vi "Event_LoadOrCreateRefs.vi"(8 "Error In":errorcluster) -> (0 "Error Out":errorcluster, 3 "HSE-Event":T1)   [LabVIEW 2014, in "hse-misc.lvlib"]
doc: "Returns the refnum of the HSE-Event\n\n\n\n____\nHAMPEL SOFTWARE ENGINEERING v0.7.0 (2018-07-16 18:12)"
uses:
  hse-misc.lvlib
  Event_GenericReference.ctl
  Event_GenericDatatype.ctl
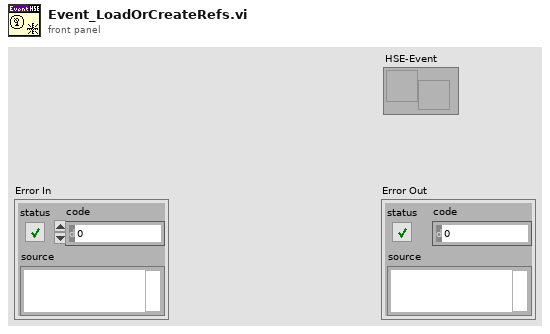
[diagram p1: front panel]
types:
  T1 = typedef "hse-misc.lvlib/Event_GenericReference.ctl" = refnum<user-event>
  T2 = typedef "hse-misc.lvlib/Event_GenericDatatype.ctl" = cluster{"name":string, "parameters":string, "data":variant}
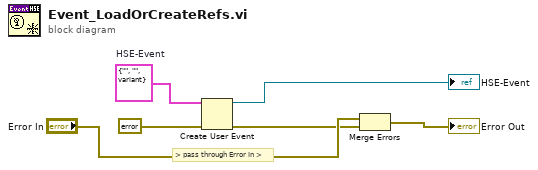
[diagram p0: block diagram]
diagram:
  w2 = T2 {"name"="", "parameters"="", "data"=variant}  # HSE-Event
  # "> pass through Error In >"
  n1 = Create User Event(user event datatype=w2, error in=errorcluster {"status"=FALSE, "code"=0, "source"=""} ("Error In")) -> (user event=→"HSE-Event":refnum<user-event>, error out=w3:errorcluster)
  n2 = Merge Errors("Error In", w3) -> (→"Error Out":errorcluster)
